vi "TestStand - Evaluate.vi"(8 "error in":errorcluster, 9 "String":string, 11 "Sequence Context":refnum<k7>) -> (0 "error out":errorcluster, 1 "Evaluate":refnum<k7>, 3 "Sequence Context":refnum<k7>)   [LabVIEW 2009]
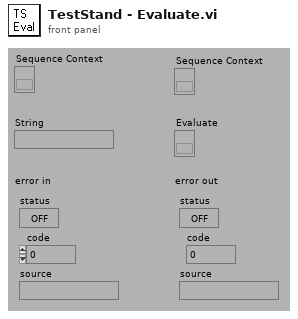
[diagram p1: front panel]
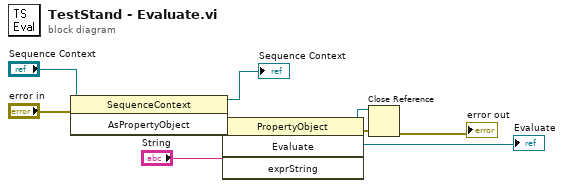
[diagram p0: block diagram]
diagram:
  n1 = invoke class="SequenceContext" method="AsPropertyObject"(reference="Sequence Context", error in="error in") -> (reference out=→"Sequence Context":refnum<k7>, error out=w5:errorcluster, "AsPropertyObject"=w1:refnum<k7>)  [unwired: 1 in]
  n2 = invoke class="PropertyObject" method="Evaluate"(reference=w1, error in=w5, "exprString"="String") -> (reference out=w8:refnum<k7>, error out=w9:errorcluster, "Evaluate"=→"Evaluate":refnum<k7>)  [unwired: 1 in, 1 out]
  n3 = Close Reference(reference=w8, error in (no error)=w9) -> (error out=→"error out":errorcluster)
